vi "uBroker_get_LastValues.vi"(6 "timeout in ms (1000)":i32=1000, 8 "error in (no error)":errorcluster, 10 "policy":refnum<class "uPolicy.lvclass">, 11 "uBroker in":refnum<class "uTransport_uActor.lvclass">) -> (0 "error out":errorcluster, 1 "Last Published Events":refnum<class "uMsg.lvclass">[](array[class]))   [LabVIEW 2023, in "uLib.lvlib" / "uBroker.lvclass"]
doc: "This is a dataflow blocking message that is used to read the last published events on all the topics that fit a specific subscription criterion."
uses:
  uBroker.lvclass
  uTransport/uTransport_uActor/uTransport_uActor.lvclass
  U:/Projects/uLib/Src/uFramework/uTransport/uTransport.lvclass
  uPolicy/uPolicy/uPolicy.lvclass
  uMsg/uMsg/uMsg.lvclass
  uData/uData/uData.lvclass
  uData/uData/uData.lvclass/uData.ctl
  uTransport/uTransport_Queue/uTransport_Queue.lvclass/uTransport_Queue.ctl
  uMsg/uMsg/uMsg.lvclass/uMsg.ctl
  uMsg/uMsg/uMsg Create.vi
  uMsg/uMsg/uMsg Get Payload.vi
  uTransport/uTransport/uTransport_SendMsg.vi
  uTransport/uTransport_Queue/uTransport_Queue_Create.vi
  uData/uData/Condition Tag Name.vi
  uMsg/uMsg/uMsg Update Timestamp.vi
  uData/uData/Blank Key Reserved String.vi
  uTransport/uTransport_Queue/uTransport_Queue.lvclass
  <vilib>/Utility/error.llb/Error Cluster From Error Code.vi
  uTransport/uTransport/uTransport.lvclass
  uBroker.lvclass/uBroker.ctl
  U:/Projects/uLib/Src/uFramework/uTransport_uActor/uTransport_uActor.lvclass
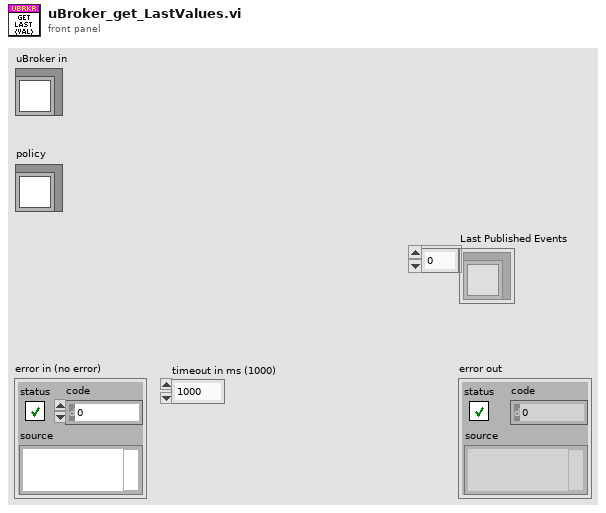
[diagram p1: front panel]
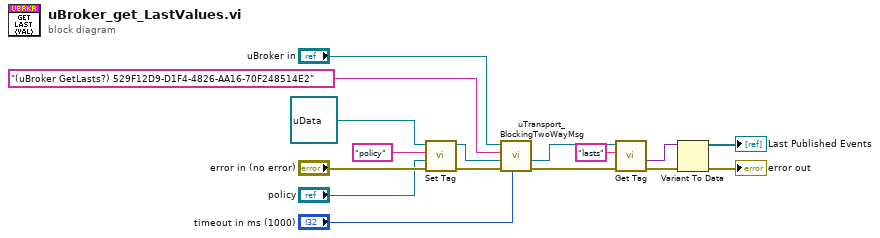
[diagram p0: block diagram]
diagram:
  n1 = call "Set Tag.vi"("error in (no error)"="error in (no error)", "Variant"="policy", "tag (case insensitive)"="policy", "uData in"=refnum<class "uData.lvclass"> refnum) -> ("error out"=w8:errorcluster, "uData out"=w7:refnum<class "uData.lvclass">)  [unwired: 5 in, 1 out]
  n2 = call "uTransport_BlockingTwoWayMsg.vi"("timeout in ms (5000)"="timeout in ms (1000)", "error in (no error)"=w8, "Data"=w7, "Command"="(uBroker GetLasts?) 529F12D9-D1F4-4826-AA16-70F248514E2", "uTransport in"="uBroker in") -> ("error out"=w13:errorcluster, "Reply"=w2:refnum<class "uData.lvclass">)  [unwired: 5 in]
  n3 = call "Get Tag.vi"("error in (no error)"=w13, "tag (case insensitive)"="lasts", "uData in"=w2) -> ("error out"=w11:errorcluster, "value"=w1:variant)  [unwired: 5 in, 2 out]
  n4 = Variant To Data(error in=w11, Variant=w1) -> (data=→"Last Published Events":refnum<class "uMsg.lvclass">[], error out=→"error out":errorcluster)  [unwired: 1 in]
